vi "Save MPLOT.vi"(8 "error in (no error)":errorcluster, 10 "RocketPlots":T1[](array[typedef]) {"RocketPlotConfig"."General"."Time to Plot" format="%<%M:%S>t"; "Plot Bounds (%)"."Bottom (%)" format="%.2f"; "Plot Bounds (%)"."Top (%)" format="%.2f"; "Plot Bounds (%)"."Right (%)" format="%.2f"; "Plot Bounds (%)"."Left (%)" format="%.2f"}, 11 "Filepath":path) -> (0 "error out":errorcluster)   [LabVIEW 2021, in "MultiRocketPlotPanel.lvclass"]
uses:
  MultiRocketPlotPanel.lvclass
  SinglePlotConfig.ctl
  SubVIs/Window Position.ctl
  <userlib>/bjustice/RocketPlot/TypeDefs/plot load data V2.ctl
  <userlib>/bjustice/RocketPlot/TypeDefs/plot properties V2.ctl
  <userlib>/bjustice/RocketPlot/TypeDefs/plot attributes V2.ctl
  <userlib>/bjustice/RocketPlot/TypeDefs/Plot scale axis properties.ctl
  <userlib>/bjustice/RocketPlot/TypeDefs/Plot general properties.ctl
  7c35f740-e301-4554-a797-b2e591fd95bb.vi
  <vilib>/JDP Science/JSONtext/Variant to JSON Text.vi
  <vilib>/JDP Science/JSONtext/LVClass Serializer/JSONtext LVClass Serializer.lvclass
  <userlib>/bjustice/RocketPlot/RocketPlot.lvlib
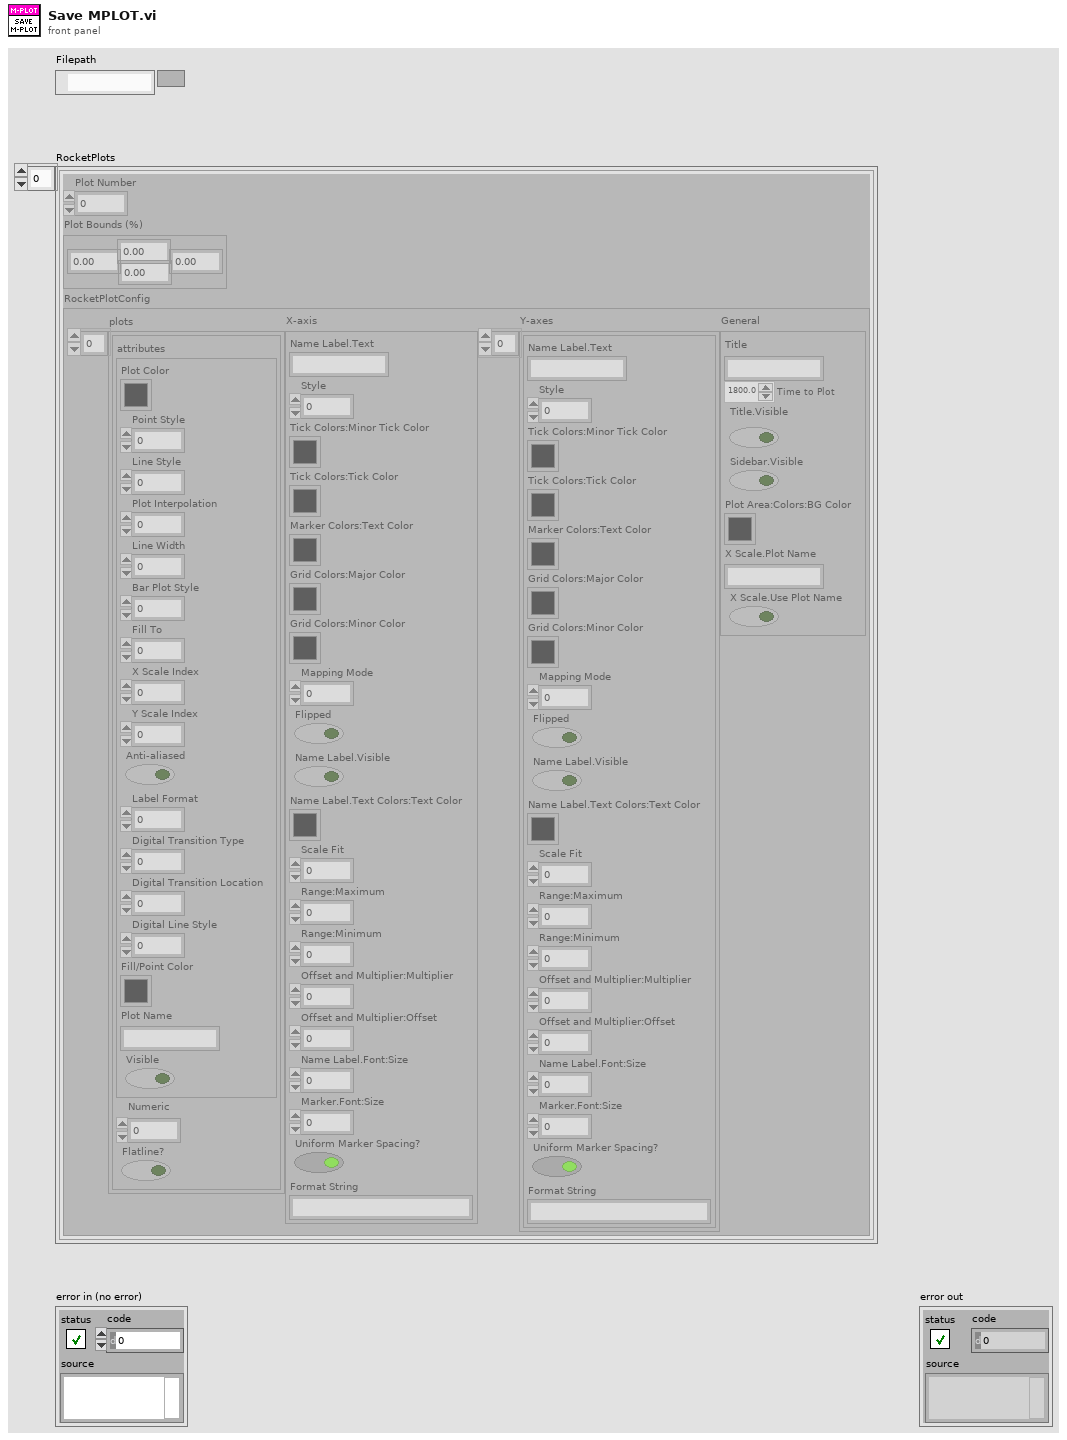
[diagram p1: front panel]
types:
  T1 = typedef "MultiRocketPlotPanel.lvclass/SinglePlotConfig.ctl" = cluster{"Plot Number":i32, "Plot Bounds (%)":T2, "RocketPlotConfig":T3}
  T2 = typedef "MultiRocketPlotPanel.lvclass/Window Position.ctl" = cluster{"Left (%)":dbl, "Top (%)":dbl, "Right (%)":dbl, "Bottom (%)":dbl}
  T3 = typedef "RocketPlot.lvlib/plot load data V2.ctl" = cluster{"plots":T4[], "X-axis":T6, "Y-axes":T6[], "General":T7}
  T4 = typedef "RocketPlot.lvlib/plot properties V2.ctl" = cluster{"attributes":T5, "Numeric":dbl, "Flatline?":bool}
  T5 = typedef "RocketPlot.lvlib/plot attributes V2.ctl" = cluster{"Plot Color":u32, "Point Style":u8, "Line Style":u8, "Plot Interpolation":u8, "Line Width":u8, "Bar Plot Style":u8, "Fill To":i16, "X Scale Index":u32, "Y Scale Index":u32, "Anti-aliased":bool, "Label Format":u8, "Digital Transition Type":u8, "Digital Transition Location":u8, "Digital Line Style":u8, "Fill/Point Color":u32, "Plot Name":string, "Visible":bool}
  T6 = typedef "RocketPlot.lvlib/Plot scale axis properties.ctl" = cluster{"Name Label.Text":string, "Style":u8, "Tick Colors:Minor Tick Color":u32, "Tick Colors:Tick Color":u32, "Marker Colors:Text Color":u32, "Grid Colors:Major Color":u32, "Grid Colors:Minor Color":u32, "Mapping Mode":u8, "Flipped":bool, "Name Label.Visible":bool, "Name Label.Text Colors:Text Color":u32, "Scale Fit":u8, "Range:Maximum":dbl, "Range:Minimum":dbl, "Offset and Multiplier:Multiplier":dbl, "Offset and Multiplier:Offset":dbl, "Name Label.Font:Size":u32, "Marker.Font:Size":u32, "Uniform Marker Spacing?":bool, "Format String":string}
  T7 = typedef "RocketPlot.lvlib/Plot general properties.ctl" = cluster{"Title":string, "Time to Plot":dbl, "Title.Visible":bool, "Sidebar.Visible":bool, "Plot Area:Colors:BG Color":u32, "X Scale.Plot Name":string, "X Scale.Use Plot Name":bool}
  T8 = enum16{"open", "replace", "create", "open or create", "replace or create", "replace or create with confirmation"}
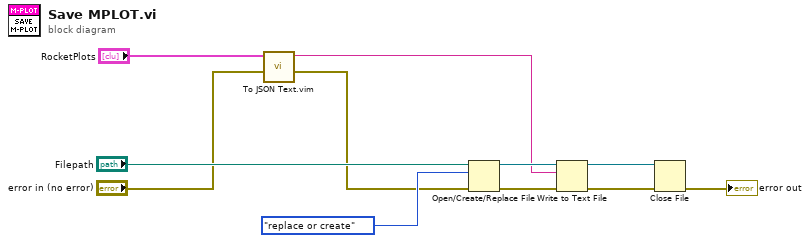
[diagram p0: block diagram]
diagram:
  n1 = call "To JSON Text.vim"("error in (no error)"="error in (no error)", "Anything"="RocketPlots") -> ("error out"=w2:errorcluster, "<JSON>"=w1:string)  [unwired: 8 in]
  n2 = Open/Create/Replace File(file path (use dialog)="Filepath", error in=w2, operation (0:open)=T8."replace or create") -> (refnum out=w10:refnum<file>, error out=w8:errorcluster)  [unwired: 3 in, 1 out]
  n3 = Write to Text File(file (use dialog)=w10, text=w1, error in=w8) -> (refnum out=w9:refnum<file>, error out=w7:errorcluster)  [unwired: 1 in, 1 out]
  n4 = Close File(refnum=w9, error in=w7) -> (error out=→"error out":errorcluster)  [unwired: 1 out]
